vi "cRIO_8maze_controls.vi"() -> ()   [LabVIEW 2019]
panel:
  out "Dzone seq.":dbl
  in  "Sound":bool
  in  "AIR_R":bool
  in  "AIR_L":bool
  out "Direction":bool[](array[boolean])
  in  "MD_R":bool
  in  "MD_L":bool
  in  "LED_R":bool
  in  "LED_L":bool
  in  "PWM rate":dbl[](array[numeric])=[0.1, 0.1, 0.1, 0.1]
  out "appended array":bool[](array[boolean])
  in  "PWM positions":dbl[](array[numeric])=[4.0, 4.4, 8.2, 9.5]
  # "Left"
  # "Right"
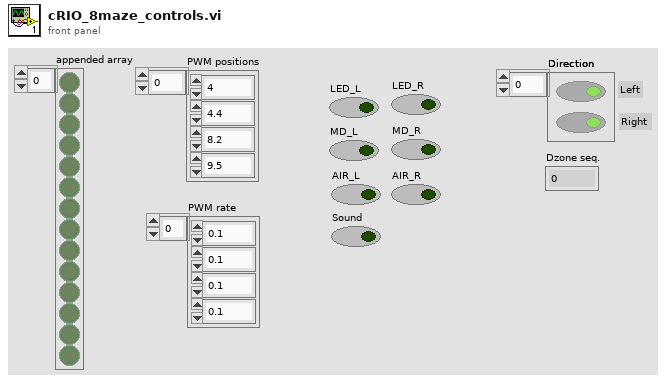
[diagram p1: front panel]
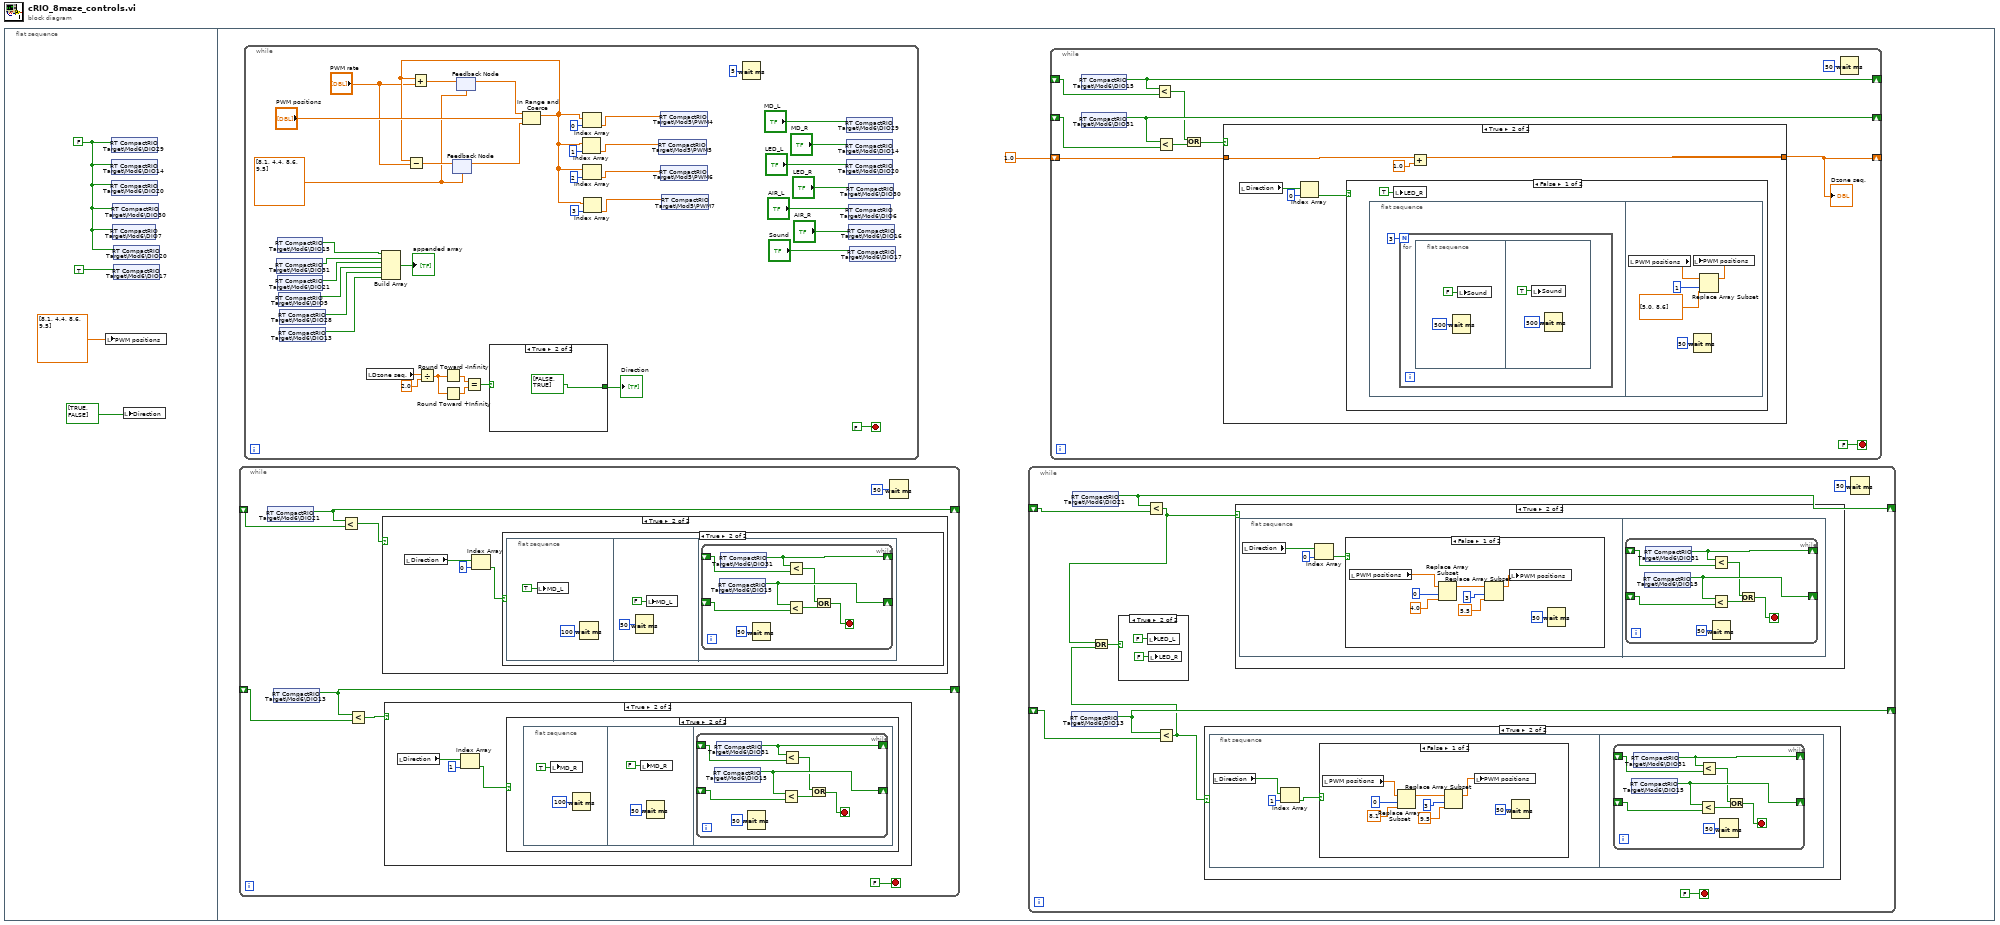
[diagram p0: block diagram]
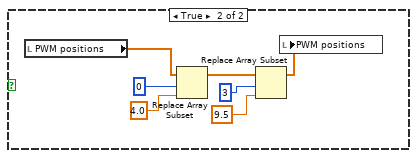
[diagram p4: hidden frame]
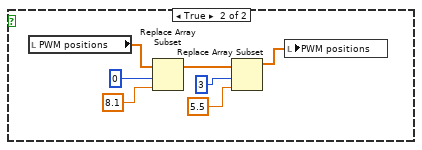
[diagram p6: hidden frame]
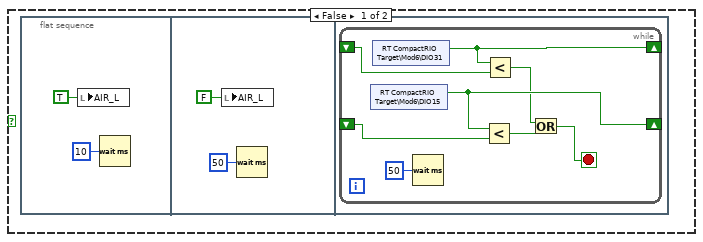
[diagram p8: hidden frame]
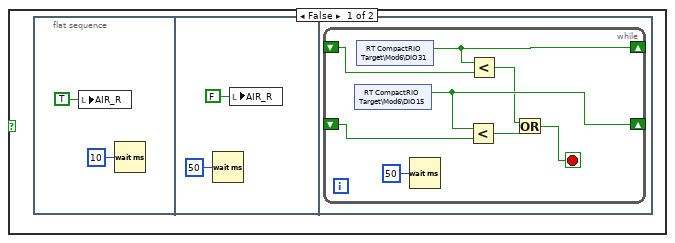
[diagram p10: hidden frame]
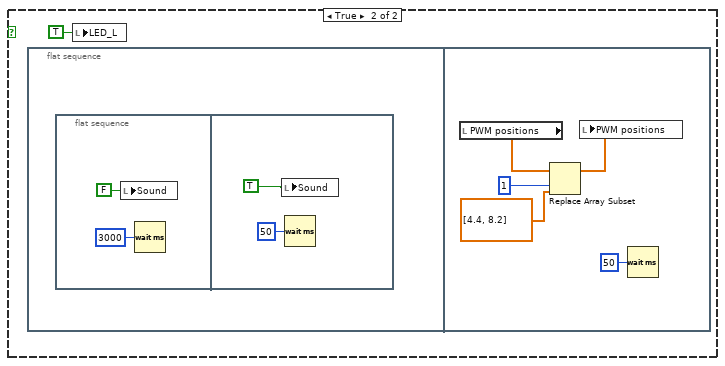
[diagram p12: hidden frame]
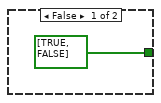
[diagram p13: hidden frame]
diagram:
  n1 = flat-sequence {
    frame #0 {
      w4 = FALSE
      n2 = local write "PWM positions"(dbl[] [8.1, 4.4, 8.6, 9.5]) -> ()
      n3 = shared-variable "RT CompactRIO Target\\Mod6\\DIO29"(w4) -> ()  [unwired: 1 in, 1 out]
      n4 = shared-variable "RT CompactRIO Target\\Mod6\\DIO14"(w4) -> ()  [unwired: 1 in, 1 out]
      n5 = shared-variable "RT CompactRIO Target\\Mod6\\DIO20"(w4) -> ()  [unwired: 1 in, 1 out]
      n6 = shared-variable "RT CompactRIO Target\\Mod6\\DIO30"(w4) -> ()  [unwired: 1 in, 1 out]
      n7 = shared-variable "RT CompactRIO Target\\Mod6\\DIO7"(w4) -> ()  [unwired: 1 in, 1 out]
      n8 = shared-variable "RT CompactRIO Target\\Mod6\\DIO20"(w4) -> ()  [unwired: 1 in, 1 out]
      n9 = shared-variable "RT CompactRIO Target\\Mod6\\DIO17"(TRUE) -> ()  [unwired: 1 in, 1 out]
      n10 = local write "Direction"(bool[] [TRUE, FALSE]) -> ()
    }
    frame #1 {
      n11 = while {
        shift-right: [w75] -> _
        shift-left: _ -> [w74]
        shift-right: [w73] -> _
        shift-left: _ -> [w72]
        stop <- FALSE stop-if-true
        n12 = shared-variable "RT CompactRIO Target\\Mod6\\DIO21"() -> (w75:bool)  [unwired: 1 in, 1 out]
        n13 = shared-variable "RT CompactRIO Target\\Mod6\\DIO13"() -> (w73:bool)  [unwired: 1 in, 1 out]
        n14 = Less?(x=w75, y=w74) -> (x < y?=w71:bool)
        n15 = Less?(x=w73, y=w72) -> (x < y?=w70:bool)
        n16 = case shown="True" w71 {
          frame False {
          }
          frame True {
            n17 = local read "Direction"() -> (w79:bool[])
            n18 = Index Array(array=w79, index=0) -> (element=w77:bool)
            n19 = case shown="True" w77 {
              frame False {
                n20 = flat-sequence {
                  frame #0 {
                    n21 = local write "AIR_L"(TRUE ("AIR_L")) -> ()
                    n22 = Wait (ms)(milliseconds to wait=u32 10) -> ()  [unwired: 1 out]
                  }
                  frame #1 {
                    n23 = local write "AIR_L"(FALSE ("AIR_R")) -> ()
                    n24 = Wait (ms)(milliseconds to wait=u32 50) -> ()  [unwired: 1 out]
                  }
                  frame #2 {
                    n25 = while {
                      shift-right: [w91] -> _
                      shift-left: _ -> [w90]
                      shift-right: [w88] -> _
                      shift-left: _ -> [w89]
                      stop <- w87 stop-if-true
                      n26 = shared-variable "RT CompactRIO Target\\Mod6\\DIO15"() -> (w91:bool)  [unwired: 1 in, 1 out]
                      n27 = shared-variable "RT CompactRIO Target\\Mod6\\DIO31"() -> (w88:bool)  [unwired: 1 in, 1 out]
                      n28 = Wait (ms)(milliseconds to wait=u32 50) -> ()  [unwired: 1 out]
                      n29 = Less?(x=w91, y=w90) -> (x < y?=w85:bool)
                      n30 = Less?(x=w88, y=w89) -> (x < y?=w86:bool)
                      n31 = Or(x=w86, y=w85) -> (x .or. y?=w87:bool)
                    }
                  }
                }
              }
              frame True {
                n32 = flat-sequence {
                  frame #0 {
                    n33 = local write "MD_L"(TRUE ("MD_L")) -> ()
                    n34 = Wait (ms)(milliseconds to wait=u32 100) -> ()  [unwired: 1 out]
                  }
                  frame #1 {
                    n35 = Wait (ms)(milliseconds to wait=u32 50) -> ()  [unwired: 1 out]
                    n36 = local write "MD_L"(FALSE ("MD_L")) -> ()
                  }
                  frame #2 {
                    n37 = while {
                      shift-right: [w103] -> _
                      shift-left: _ -> [w102]
                      shift-right: [w100] -> _
                      shift-left: _ -> [w101]
                      stop <- w99 stop-if-true
                      n38 = shared-variable "RT CompactRIO Target\\Mod6\\DIO15"() -> (w103:bool)  [unwired: 1 in, 1 out]
                      n39 = shared-variable "RT CompactRIO Target\\Mod6\\DIO31"() -> (w100:bool)  [unwired: 1 in, 1 out]
                      n40 = Wait (ms)(milliseconds to wait=u32 50) -> ()  [unwired: 1 out]
                      n41 = Less?(x=w103, y=w102) -> (x < y?=w97:bool)
                      n42 = Less?(x=w100, y=w101) -> (x < y?=w98:bool)
                      n43 = Or(x=w98, y=w97) -> (x .or. y?=w99:bool)
                    }
                  }
                }
              }
            }
          }
        }
        n44 = case shown="True" w70 {
          frame False {
          }
          frame True {
            n45 = local read "Direction"() -> (w106:bool[])
            n46 = Index Array(array=w106, index=1) -> (element=w104:bool)
            n47 = case shown="True" w104 {
              frame False {
                n48 = flat-sequence {
                  frame #0 {
                    n49 = local write "AIR_R"(TRUE ("AIR_R")) -> ()
                    n50 = Wait (ms)(milliseconds to wait=u32 10) -> ()  [unwired: 1 out]
                  }
                  frame #1 {
                    n51 = Wait (ms)(milliseconds to wait=u32 50) -> ()  [unwired: 1 out]
                    n52 = local write "AIR_R"(FALSE ("AIR_R")) -> ()
                  }
                  frame #2 {
                    n53 = while {
                      shift-right: [w118] -> _
                      shift-left: _ -> [w117]
                      shift-right: [w115] -> _
                      shift-left: _ -> [w116]
                      stop <- w114 stop-if-true
                      n54 = shared-variable "RT CompactRIO Target\\Mod6\\DIO15"() -> (w118:bool)  [unwired: 1 in, 1 out]
                      n55 = shared-variable "RT CompactRIO Target\\Mod6\\DIO31"() -> (w115:bool)  [unwired: 1 in, 1 out]
                      n56 = Wait (ms)(milliseconds to wait=u32 50) -> ()  [unwired: 1 out]
                      n57 = Less?(x=w118, y=w117) -> (x < y?=w112:bool)
                      n58 = Less?(x=w115, y=w116) -> (x < y?=w113:bool)
                      n59 = Or(x=w113, y=w112) -> (x .or. y?=w114:bool)
                    }
                  }
                }
              }
              frame True {
                n60 = flat-sequence {
                  frame #0 {
                    n61 = local write "MD_R"(TRUE ("MD_R")) -> ()
                    n62 = Wait (ms)(milliseconds to wait=u32 100) -> ()  [unwired: 1 out]
                  }
                  frame #1 {
                    n63 = local write "MD_R"(FALSE ("MD_R")) -> ()
                    n64 = Wait (ms)(milliseconds to wait=u32 50) -> ()  [unwired: 1 out]
                  }
                  frame #2 {
                    n65 = while {
                      shift-right: [w130] -> _
                      shift-left: _ -> [w129]
                      shift-right: [w127] -> _
                      shift-left: _ -> [w128]
                      stop <- w126 stop-if-true
                      n66 = shared-variable "RT CompactRIO Target\\Mod6\\DIO15"() -> (w130:bool)  [unwired: 1 in, 1 out]
                      n67 = shared-variable "RT CompactRIO Target\\Mod6\\DIO31"() -> (w127:bool)  [unwired: 1 in, 1 out]
                      n68 = Wait (ms)(milliseconds to wait=u32 50) -> ()  [unwired: 1 out]
                      n69 = Less?(x=w130, y=w129) -> (x < y?=w124:bool)
                      n70 = Less?(x=w127, y=w128) -> (x < y?=w125:bool)
                      n71 = Or(x=w125, y=w124) -> (x .or. y?=w126:bool)
                    }
                  }
                }
              }
            }
          }
        }
        n72 = Wait (ms)(milliseconds to wait=u32 50) -> ()  [unwired: 1 out]
      }
      n73 = while {
        stop <- FALSE stop-if-true
        w192 = dbl[] [8.1, 4.4, 8.6, 9.5]
        n74 = shared-variable "RT CompactRIO Target\\Mod6\\DIO31"() -> (w180:bool)  [unwired: 1 in, 1 out]
        n75 = shared-variable "RT CompactRIO Target\\Mod6\\DIO15"() -> (w186:bool)  [unwired: 1 in, 1 out]
        n76 = shared-variable "RT CompactRIO Target\\Mod6\\DIO21"() -> (w181:bool)  [unwired: 1 in, 1 out]
        n77 = shared-variable "RT CompactRIO Target\\Mod6\\DIO5"() -> (w182:bool)  [unwired: 1 in, 1 out]
        n78 = shared-variable "RT CompactRIO Target\\Mod6\\DIO28"() -> (w183:bool)  [unwired: 1 in, 1 out]
        n79 = shared-variable "RT CompactRIO Target\\Mod6\\DIO13"() -> (w184:bool)  [unwired: 1 in, 1 out]
        n80 = local read "Dzone seq."() -> (w176:dbl)
        n81 = Build Array(w186, w180, w181, w182, w183, w184) -> (→"appended array":bool[])
        n82 = Divide(x=w176, y=2.0) -> (x/y=w174:dbl)
        n83 = Round Toward -Infinity(1:w174) -> (0:w173:dbl)
        n84 = Round Toward +Infinity(x=w174) -> (ceil(x): smallest int >= x=w172:dbl)
        n85 = feedback #1(w192) -> (w193:dbl[])
        n86 = feedback #2(w192) -> (w196:dbl[])
        n87 = Equal?(x=w173, y=w172) -> (x = y?=w171:bool)
        n88 = case shown="True" w171 {
          tunnel: [bool[] [TRUE, FALSE] bool[] [FALSE, TRUE]] -> w170
          frame False {
          }
          frame True {
          }
        }
        "Direction" <- w170
        n89 = In Range and Coerce(upper limit=w196, x="PWM positions", lower limit=w193) -> (coerced(x)=w195:dbl[])  [unwired: 1 out]
        n90 = Subtract(x=w195, y="PWM rate") -> (x-y=w194:dbl[])
        n91 = Add(x=w195, y="PWM rate") -> (x+y=w197:dbl[])
        n92 = feedback-in #1(w194) -> ()
        n93 = feedback-in #2(w197) -> ()
        n94 = Index Array(array=w195, index=1) -> (element=w206:dbl)
        n95 = Index Array(array=w195, index=0) -> (element=w205:dbl)
        n96 = Index Array(array=w195, index=2) -> (element=w207:dbl)
        n97 = Index Array(array=w195, index=3) -> (element=w208:dbl)
        n98 = shared-variable "RT CompactRIO Target\\Mod5\\PWM5"(w206) -> ()  [unwired: 1 in, 1 out]
        n99 = shared-variable "RT CompactRIO Target\\Mod5\\PWM4"(w205) -> ()  [unwired: 1 in, 1 out]
        n100 = shared-variable "RT CompactRIO Target\\Mod5\\PWM6"(w207) -> ()  [unwired: 1 in, 1 out]
        n101 = shared-variable "RT CompactRIO Target\\Mod5\\PWM7"(w208) -> ()  [unwired: 1 in, 1 out]
        n102 = Wait (ms)(milliseconds to wait=u32 5) -> ()  [unwired: 1 out]
        n103 = shared-variable "RT CompactRIO Target\\Mod6\\DIO29"("MD_L") -> ()  [unwired: 1 in, 1 out]
        n104 = shared-variable "RT CompactRIO Target\\Mod6\\DIO14"("MD_R") -> ()  [unwired: 1 in, 1 out]
        n105 = shared-variable "RT CompactRIO Target\\Mod6\\DIO20"("LED_L") -> ()  [unwired: 1 in, 1 out]
        n106 = shared-variable "RT CompactRIO Target\\Mod6\\DIO30"("LED_R") -> ()  [unwired: 1 in, 1 out]
        n107 = shared-variable "RT CompactRIO Target\\Mod6\\DIO6"("AIR_L") -> ()  [unwired: 1 in, 1 out]
        n108 = shared-variable "RT CompactRIO Target\\Mod6\\DIO16"("AIR_R") -> ()  [unwired: 1 in, 1 out]
        n109 = shared-variable "RT CompactRIO Target\\Mod6\\DIO17"("Sound") -> ()  [unwired: 1 in, 1 out]
      }
      n110 = while {
        shift-right: [w9] -> _
        shift-left: _ -> [w12]
        shift-right: [w10] -> _
        shift-left: _ -> [w11]
        stop <- FALSE stop-if-true
        n111 = shared-variable "RT CompactRIO Target\\Mod6\\DIO13"() -> (w10:bool)  [unwired: 1 in, 1 out]
        n112 = shared-variable "RT CompactRIO Target\\Mod6\\DIO21"() -> (w9:bool)  [unwired: 1 in, 1 out]
        n113 = Less?(x=w9, y=w12) -> (x < y?=w7:bool)
        n114 = Less?(x=w10, y=w11) -> (x < y?=w6:bool)
        n115 = Or(x=w7, y=w6) -> (x .or. y?=w8:bool)
        n116 = case shown="True" w8 {
          frame False {
          }
          frame True {
            n117 = local write "LED_L"(FALSE ("LED_L")) -> ()
            n118 = local write "LED_R"(FALSE ("LED_R")) -> ()
          }
        }
        n119 = case shown="True" w6 {
          frame False {
          }
          frame True {
            n120 = flat-sequence {
              frame #0 {
                n121 = local read "Direction"() -> (w18:bool[])
                n122 = Index Array(array=w18, index=1) -> (element=w17:bool)
                n123 = case shown="False" w17 {
                  frame False {
                    n124 = local read "PWM positions"() -> (w23:dbl[])
                    n125 = Replace Array Subset(array=w23, new element=8.1 ("new element/subarray"), index=0) -> (w22:dbl[])
                    n126 = Replace Array Subset(array=w22, new element=9.5 ("new element/subarray"), index=3) -> (w21:dbl[])
                    n127 = local write "PWM positions"(w21) -> ()
                    n128 = Wait (ms)(milliseconds to wait=u32 50) -> ()  [unwired: 1 out]
                  }
                  frame True {
                    n129 = local read "PWM positions"() -> (w30:dbl[])
                    n130 = Replace Array Subset(array=w30, new element=4.0 ("new element/subarray"), index=0) -> (w28:dbl[])
                    n131 = Replace Array Subset(array=w28, new element=9.5 ("new element/subarray"), index=3) -> (w29:dbl[])
                    n132 = local write "PWM positions"(w29) -> ()
                  }
                }
              }
              frame #1 {
                n133 = while {
                  shift-right: [w42] -> _
                  shift-left: _ -> [w41]
                  shift-right: [w39] -> _
                  shift-left: _ -> [w40]
                  stop <- w38 stop-if-true
                  n134 = shared-variable "RT CompactRIO Target\\Mod6\\DIO15"() -> (w42:bool)  [unwired: 1 in, 1 out]
                  n135 = shared-variable "RT CompactRIO Target\\Mod6\\DIO31"() -> (w39:bool)  [unwired: 1 in, 1 out]
                  n136 = Less?(x=w42, y=w41) -> (x < y?=w36:bool)
                  n137 = Less?(x=w39, y=w40) -> (x < y?=w37:bool)
                  n138 = Wait (ms)(milliseconds to wait=u32 50) -> ()  [unwired: 1 out]
                  n139 = Or(x=w37, y=w36) -> (x .or. y?=w38:bool)
                }
              }
            }
          }
        }
        n140 = case shown="True" w7 {
          frame False {
          }
          frame True {
            n141 = flat-sequence {
              frame #0 {
                n142 = local read "Direction"() -> (w44:bool[])
                n143 = Index Array(array=w44, index=0) -> (element=w43:bool)
                n144 = case shown="False" w43 {
                  frame False {
                    n145 = local read "PWM positions"() -> (w48:dbl[])
                    n146 = Replace Array Subset(array=w48, new element=4.0 ("new element/subarray"), index=0) -> (w49:dbl[])
                    n147 = Replace Array Subset(array=w49, new element=5.5 ("new element/subarray"), index=3) -> (w47:dbl[])
                    n148 = local write "PWM positions"(w47) -> ()
                    n149 = Wait (ms)(milliseconds to wait=u32 50) -> ()  [unwired: 1 out]
                  }
                  frame True {
                    n150 = local read "PWM positions"() -> (w60:dbl[])
                    n151 = Replace Array Subset(array=w60, new element=8.1 ("new element/subarray"), index=0) -> (w55:dbl[])
                    n152 = Replace Array Subset(array=w55, new element=5.5 ("new element/subarray"), index=3) -> (w54:dbl[])
                    n153 = local write "PWM positions"(w54) -> ()
                  }
                }
              }
              frame #1 {
                n154 = while {
                  shift-right: [w68] -> _
                  shift-left: _ -> [w67]
                  shift-right: [w65] -> _
                  shift-left: _ -> [w66]
                  stop <- w64 stop-if-true
                  n155 = shared-variable "RT CompactRIO Target\\Mod6\\DIO15"() -> (w68:bool)  [unwired: 1 in, 1 out]
                  n156 = shared-variable "RT CompactRIO Target\\Mod6\\DIO31"() -> (w65:bool)  [unwired: 1 in, 1 out]
                  n157 = Less?(x=w68, y=w67) -> (x < y?=w62:bool)
                  n158 = Less?(x=w65, y=w66) -> (x < y?=w63:bool)
                  n159 = Wait (ms)(milliseconds to wait=u32 50) -> ()  [unwired: 1 out]
                  n160 = Or(x=w63, y=w62) -> (x .or. y?=w64:bool)
                }
              }
            }
          }
        }
        n161 = Wait (ms)(milliseconds to wait=u32 50) -> ()  [unwired: 1 out]
      }
      n162 = while {
        shift-right: [w141] -> _
        shift-left: _ -> [w140]
        shift-right: [w138] -> _
        shift-left: _ -> [w139]
        shift-right: [w132] -> _
        shift-left: 1.0 -> [w131]
        stop <- FALSE stop-if-true
        n163 = shared-variable "RT CompactRIO Target\\Mod6\\DIO15"() -> (w141:bool)  [unwired: 1 in, 1 out]
        n164 = shared-variable "RT CompactRIO Target\\Mod6\\DIO31"() -> (w138:bool)  [unwired: 1 in, 1 out]
        n165 = Less?(x=w141, y=w140) -> (x < y?=w134:bool)
        n166 = Less?(x=w138, y=w139) -> (x < y?=w135:bool)
        n167 = Or(x=w134, y=w135) -> (x .or. y?=w133:bool)
        n168 = case shown="True" w133 {
          tunnel: [w142 w145] -> w132
          tunnel: w131 -> [w142 w143]
          frame False {
          }
          frame True {
            n169 = local read "Direction"() -> (w148:bool[])
            n170 = Index Array(array=w148, index=0) -> (element=w146:bool)
            n171 = case shown="False" w146 {
              frame False {
                n172 = flat-sequence {
                  frame #0 {
                    n173 = for {
                      N: 3 -> [_]
                      n174 = flat-sequence {
                        frame #0 {
                          n175 = Wait (ms)(milliseconds to wait=u32 500) -> ()  [unwired: 1 out]
                          n176 = local write "Sound"(FALSE ("Sound")) -> ()
                        }
                        frame #1 {
                          n177 = local write "Sound"(TRUE ("Sound")) -> ()
                          n178 = Wait (ms)(milliseconds to wait=u32 500) -> ()  [unwired: 1 out]
                        }
                      }
                    }
                  }
                  frame #1 {
                    n179 = local read "PWM positions"() -> (w159:dbl[])
                    n180 = Wait (ms)(milliseconds to wait=u32 50) -> ()  [unwired: 1 out]
                    n181 = Replace Array Subset(array=w159, new element=dbl[] [5.0, 8.6] ("new element/subarray"), index=1) -> (w156:dbl[])
                    n182 = local write "PWM positions"(w156) -> ()
                  }
                }
                n183 = local write "LED_R"(TRUE ("LED_R")) -> ()
              }
              frame True {
                n184 = flat-sequence {
                  frame #0 {
                    n185 = flat-sequence {
                      frame #0 {
                        n186 = local write "Sound"(FALSE ("Sound")) -> ()
                        n187 = Wait (ms)(milliseconds to wait=u32 3000) -> ()  [unwired: 1 out]
                      }
                      frame #1 {
                        n188 = local write "Sound"(TRUE ("LED_L")) -> ()
                        n189 = Wait (ms)(milliseconds to wait=u32 50) -> ()  [unwired: 1 out]
                      }
                    }
                  }
                  frame #1 {
                    n190 = local read "PWM positions"() -> (w167:dbl[])
                    n191 = Replace Array Subset(array=w167, new element=dbl[] [4.4, 8.2] ("new element/subarray"), index=1) -> (w166:dbl[])
                    n192 = local write "PWM positions"(w166) -> ()
                    n193 = Wait (ms)(milliseconds to wait=u32 50) -> ()  [unwired: 1 out]
                  }
                }
                n194 = local write "LED_L"(TRUE ("LED_L")) -> ()
              }
            }
            n195 = Add(x=w143, y=1.0) -> (x+y=w145:dbl)
          }
        }
        "Dzone seq." <- w132
        n196 = Wait (ms)(milliseconds to wait=u32 50) -> ()  [unwired: 1 out]
      }
    }
  }
